vi "Load All Firmware Config Data.vi"(8 "Error In":errorcluster) -> (0 "Error Out":errorcluster, 1 "Firmwares":T2[][][](array[typedef]), 2 "Devices":T1[][](array[typedef]), 3 "Families":string[](array[string]))   [LabVIEW 2020, in "LMH-LINX.lvlib"]
uses:
  LMH-LINX.lvlib
  Type Defs/Device Firmware.ctl
  Type Defs/Device Data.ctl
  Type Defs/All Firmware Data FGV States.ctl
  Toolbox/LMH-Toolbox.lvlib
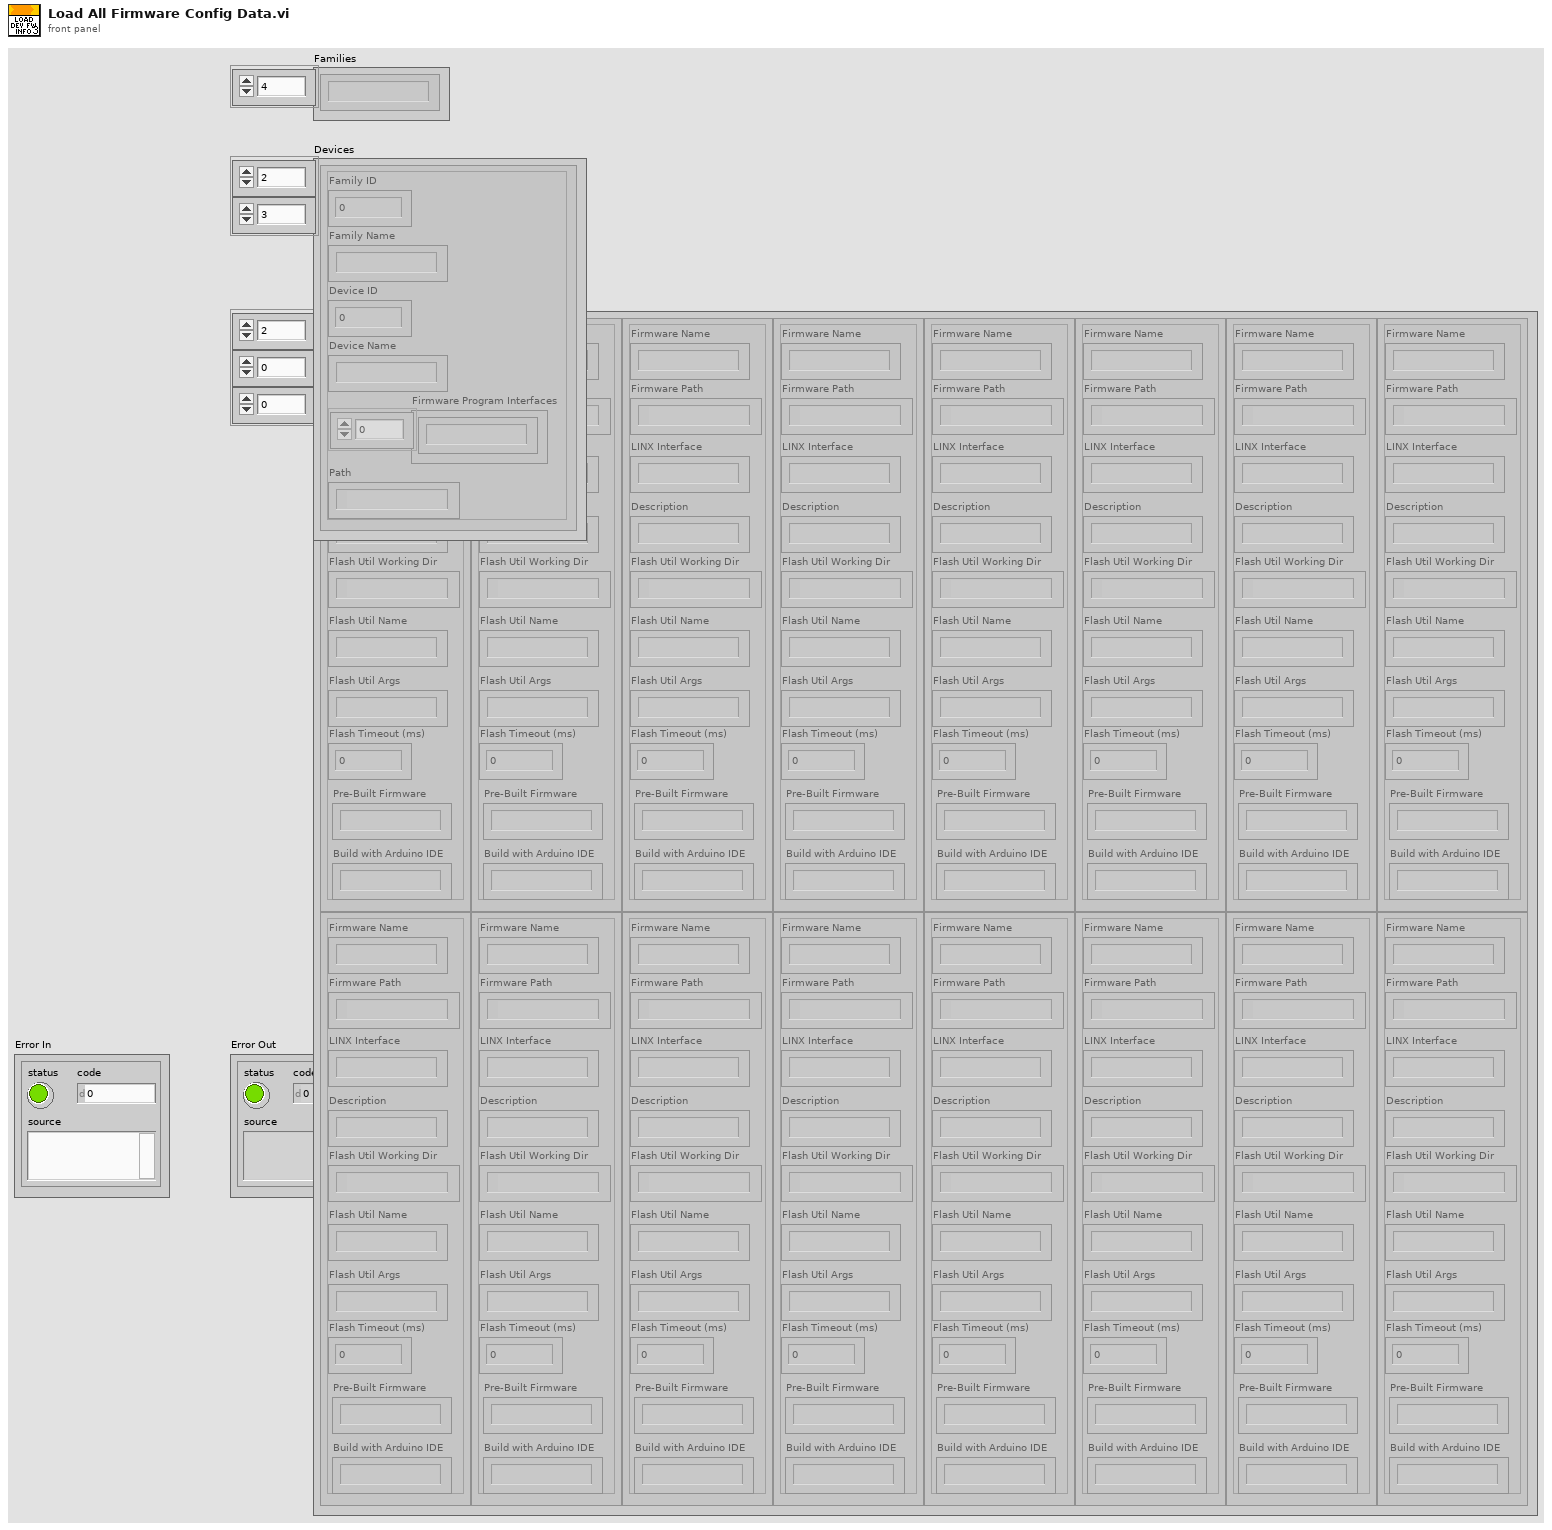
[diagram p1: front panel]
types:
  T1 = typedef "LMH-LINX.lvlib/Device Data.ctl" = cluster{"Family ID":i32, "Family Name":string, "Device ID":i32, "Device Name":string, "Firmware Program Interfaces":string[], "Path":path}
  T2 = typedef "LMH-LINX.lvlib/Device Firmware.ctl" = cluster{"Firmware Name":string, "Firmware Path":path, "Description":string, "LINX Interface":string, "Flash Util Working Dir":path, "Flash Util Name":string, "Flash Util Args":string, "Flash Timeout (ms)":i32, "Pre-Built Firmware":string, "Build with Arduino IDE":string}
  T3 = typedef "LMH-LINX.lvlib/All Firmware Data FGV States.ctl" = enum16{"Set", "Get"}
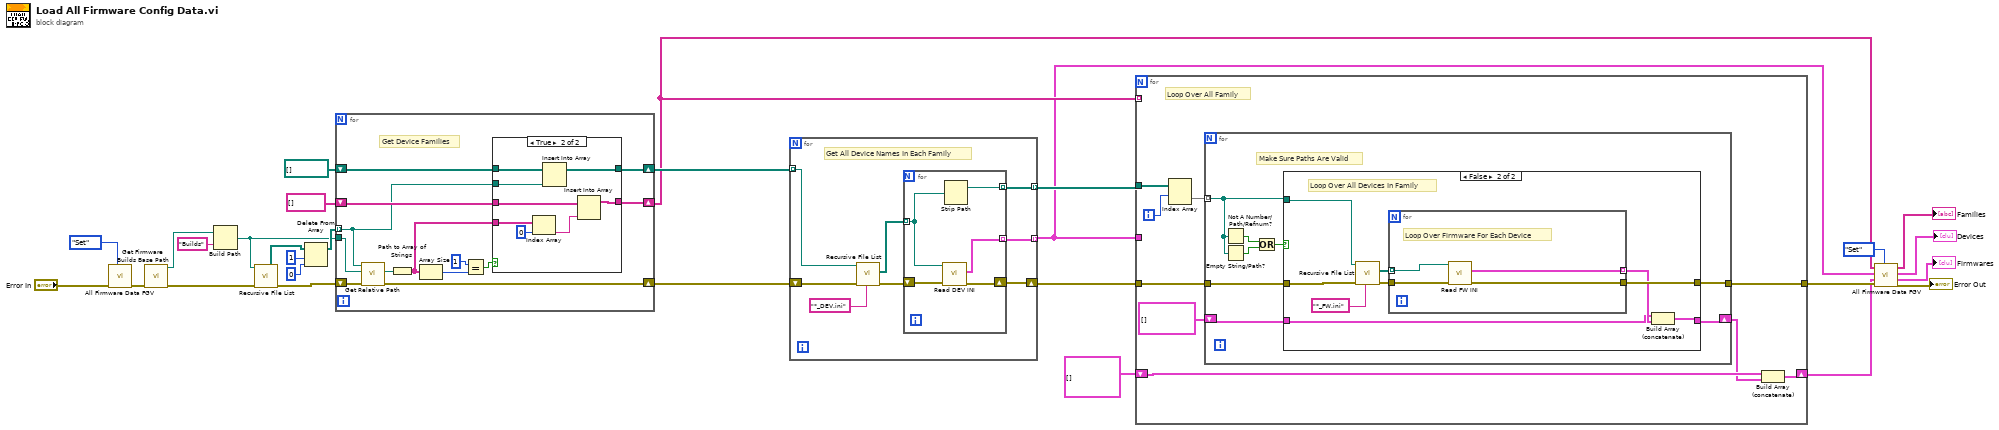
[diagram p0: block diagram]
diagram:
  n1 = call "All Firmware Data FGV.vi"("All Firmware Data FGV States"=All_Firmware_Data_FGV_States."Set", "Error In"="Error In") -> ("Error Out"=w5:errorcluster)  [unwired: 6 in, 3 out]
  n2 = call "Get Firmware Builds Base Path.vi"("Error In"=w5) -> ("Error Out"=w28:errorcluster, "Firmware Builds Base Path"=w8:path)  [unwired: 9 in]
  n3 = Build Path(base path=w8, name or relative path="Builds") -> (appended path=w6:path)
  n4 = call <vilib>:"Recursive File List.vi"("error in (no error)"=w28, "Folder Path"=w6) -> ("error out"=w27:errorcluster, "All Folders"=w24:path[])  [unwired: 5 in, 3 out]
  n5 = Delete From Array(array=w24, length=1 ("index"), index=0) -> (array with subset deleted=w23:path[])  [unwired: 1 out]
  n6 = for {
    tunnel: w23 -> [w31] mode=indexing
    tunnel: w6 -> [w32]
    shift-right: [w34] -> w14
    shift-left: string[] [] -> [w33]
    shift-right: [w40] -> w19
    shift-left: w27 -> [w41]
    shift-right: [w30] -> w20
    shift-left: path[] [] -> [w29]
    # "Get Device Families"
    n7 = call "Get Relative Path.vi"("Error In"=w41, "Relative Path Root"=w32, "File / Folder"=w31) -> ("Error Out"=w40:errorcluster, "Relative Path"=w39:path)  [unwired: 6 in, 1 out]
    n8 = Path to Array of Strings(0:w39) -> (2:w35:string[])  [unwired: 1 out]
    n9 = Array Size(array=w35) -> (size(s)=w38:i32)
    n10 = Equal?(x=1, y=w38) -> (x = y?=w36:bool)
    n11 = case shown="True" w36 {
      tunnel: w35 -> [_ w51]
      tunnel: [w43 w48] -> w34
      tunnel: w33 -> [w43 w49]
      tunnel: w31 -> [_ w45]
      tunnel: [w42 w46] -> w30
      tunnel: w29 -> [w42 w44]
      frame False {
      }
      frame True {
        n12 = Index Array(array=w51, index=0) -> (element=w47:string)
        n13 = Insert Into Array(array=w44, new element=w45) -> (w46:path[])  [unwired: 1 in]
        n14 = Insert Into Array(array=w49, new element=w47) -> (w48:string[])  [unwired: 1 in]
      }
    }
  }
  n15 = for {
    tunnel: w20 -> [w59] mode=indexing
    tunnel: [w54] -> w12 mode=indexing
    shift-right: [w53] -> w18
    shift-left: w19 -> [w58]
    tunnel: [w52] -> w17 mode=indexing
    # "Get All Device Names In Each Family"
    n16 = call <vilib>:"Recursive File List.vi"("pattern"="*_DEV.ini", "error in (no error)"=w58, "Folder Path"=w59) -> ("error out"=w55:errorcluster, "All Files in Dir"=w56:path[])  [unwired: 4 in, 3 out]
    n17 = for {
      tunnel: w56 -> [w61] mode=indexing
      tunnel: [w60] -> w54 mode=indexing
      shift-right: [w62] -> w53
      shift-left: w55 -> [w63]
      tunnel: [w64] -> w52 mode=indexing
      n18 = call "Read DEV INI.vi"("Error In"=w63, "Firmware INI Path"=w61) -> ("Error Out"=w62:errorcluster, "Device Data"=w60:T1)  [unwired: 7 in, 1 out]
      n19 = Strip Path(path=w61) -> (stripped path=w64:path)  [unwired: 1 out]
    }
  }
  n20 = for {
    tunnel: w12 -> [_]
    tunnel: w18 -> [w69]
    tunnel: [w72] -> w16
    tunnel: w17 -> [w70]
    tunnel: w14 -> [_] mode=indexing
    shift-right: [w66] -> w1
    shift-left: T2[][][] [] -> [w67]
    i -> [w73]
    # "Loop Over All Family"
    n21 = Index Array(array=w70, index (row)=w73) -> (element=w71:path[])  [unwired: 1 in]
    n22 = for {
      tunnel: [w81] -> w72
      tunnel: w71 -> [w76] mode=indexing
      tunnel: w69 -> [w80]
      shift-right: [w75] -> w65
      shift-left: T2[][] [] -> [w74]
      # "Make Sure Paths Are Valid"
      n23 = Not A Number/Path/Refnum?(number/path/refnum=w76) -> (NaN/Path/Refnum?=w79:bool)
      n24 = Empty String/Path?(string/path=w76) -> (empty?=w78:bool)
      n25 = Or(x=w79, y=w78) -> (x .or. y?=w77:bool)
      n26 = case shown="False" w77 {
        tunnel: [w83 w92] -> w81
        tunnel: w80 -> [w83 w90]
        tunnel: w76 -> [_ w89]
        tunnel: [w82 w86] -> w75
        tunnel: w74 -> [w82 w84]
        frame True {
          # "Bad Path, Skip It"
        }
        frame False {
          # "Loop Over All Devices In Family"
          n27 = call <vilib>:"Recursive File List.vi"("pattern"="*_FW.ini", "error in (no error)"=w90, "Folder Path"=w89) -> ("error out"=w87:errorcluster, "All Files in Dir"=w88:path[])  [unwired: 4 in, 3 out]
          n28 = for {
            tunnel: [w96] -> w92
            tunnel: [w95] -> w85 mode=indexing
            tunnel: w88 -> [w94] mode=indexing
            tunnel: w87 -> [w93]
            # "Loop Over Firmware For Each Device"
            n29 = call "Read FW INI.vi"("Error In"=w93, "Firmware INI Path"=w94) -> ("Error Out"=w96:errorcluster, "Firmware Config"=w95:T2)  [unwired: 7 in, 1 out]
          }
          n30 = Build Array (concatenate)(w84, w85) -> (w86:T2[][])
        }
      }
    }
    n31 = Build Array (concatenate)(w67, w65) -> (w66:T2[][][])
  }
  n32 = call "All Firmware Data FGV.vi"("All Firmware Data FGV States"=All_Firmware_Data_FGV_States."Set", "Error In"=w16, "Firmwares"=w1, "Devices"=w12, "Families"=w14) -> ("Error Out"=→"Error Out":errorcluster, "Firmwares"=→"Firmwares":T2[][][], "Devices"=→"Devices":T1[][], "Families"=→"Families":string[])  [unwired: 3 in]
